vi "InitializeViewPrototype.vi"(8 "error in (no error)":errorcluster, 11 "ViewMgr in":refnum<class "ViewMgr.lvclass">) -> (0 "error out":errorcluster, 3 "ViewMgr out":refnum<class "ViewMgr.lvclass">)   [LabVIEW 2020, in "CSM-TagDBDisplayContainer.lvlib" / "ViewMgr.lvclass"]
uses:
  ViewMgr.lvclass
  ViewMgr.lvclass/ViewMgr.ctl
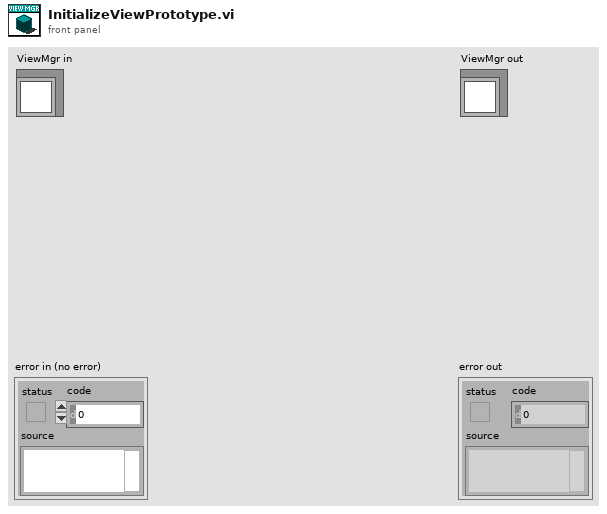
[diagram p1: front panel]
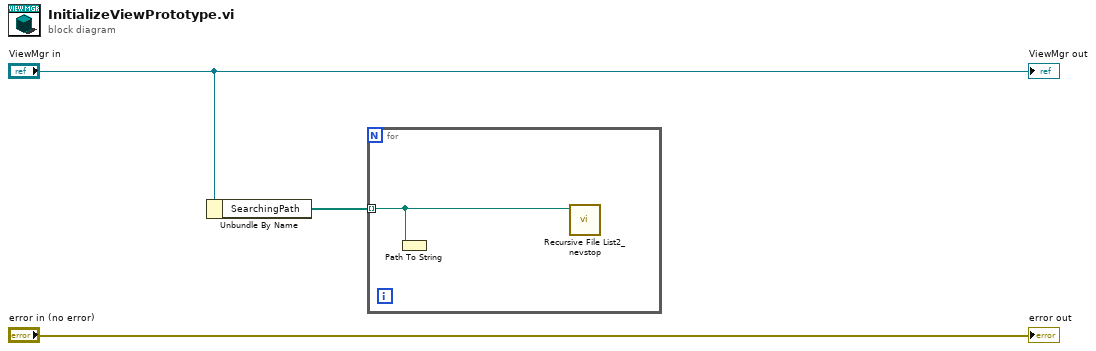
[diagram p0: block diagram]
diagram:
  n1 = Unbundle By Name("ViewMgr in") -> ("SearchingPath"=w1:path[])
  n2 = for {
    tunnel: w1 -> [w4] mode=indexing
    n3 = Path To String(path=w4) -> ()  [unwired: 1 out]
    n4 = call <userlib>:"Recursive File List2_nevstop.vi"("Folder Path"=w4) -> ()  [unwired: 6 in, 5 out]
  }
  "error out" <- "error in (no error)"
  "ViewMgr out" <- "ViewMgr in"
